vi "fxpAvgSCTL.vi"(7 "reset":bool, 8 "clear":bool, 10 "inputValid":bool=TRUE, 11 "input":fxp<+/-,16,1>) -> (0 "outputValid":bool, 2 "noAvg":u16, 3 "average":fxp<+/-,22,1>, 6 "readyForInput":bool)   [LabVIEW 2016]
uses:
  <vilib>/rvi/FXPMathLib/FxpDiv/subVIs/nifxpmath_Div_SimConfig.ctl
  <vilib>/rvi/FXPMathLib/FxpDiv/simVIs/DllFxpDivTemp_sub.vi
  <vilib>/rvi/FXPMathLib/FxpDiv/XNode/nifxpmath_Div.xnode
  <vilib>/rvi/FXPMathLib/FxpAdd/XNode/nifxpmath_Add.xnode
  <vilib>/rvi/FXPMathLib/sim/FxpSim.dll
panel:
  out "x+y":fxp<+/-,38,16>
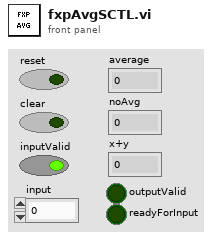
[diagram p1: front panel]
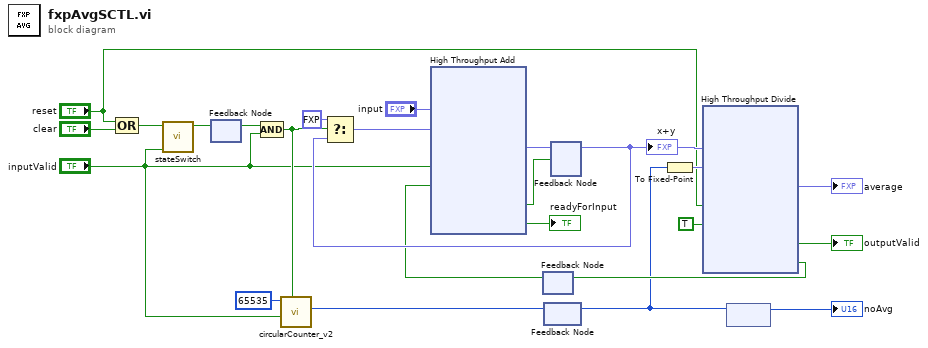
[diagram p0: block diagram]
diagram:
  n1 = Compound Arithmetic op=OR("reset", "clear") -> (w6:bool)
  n2 = call "stateSwitch.vi"("disable"="inputValid", "enable"=w6) -> ("state"=w19:bool)  [unwired: 9 in]
  n3 = feedback #1() -> (w5:bool)  [unwired: 1 in]
  n4 = feedback-in #1(w19) -> ()
  n5 = Compound Arithmetic op=AND(w5, "inputValid") -> (w7:bool)
  n6 = call "circularCounter_v2.vi"("reset"=w7, "doStep"="inputValid", "maxCount"=u16 65535) -> ("next"=w23:u16)  [unwired: 5 in, 3 out]
  n7 = feedback #2() -> (w4:bool)  [unwired: 1 in]
  n8 = feedback #3() -> (w14:u16)  [unwired: 1 in]
  n9 = feedback-in #3(w23) -> ()
  n10 = feedback #4() -> (w13:fxp<+/-,38,16>)  [unwired: 1 in]
  "x+y" <- w13
  n11 = Select(t=fxp<+/-,38,16> 0.0, s=w7, f=w13) -> (s? t:f=w18:fxp<+/-,38,16>)
  n12 = xnode ("High Throughput Add")("x"="input", "y"=w18, "input valid"="inputValid", "ready for output (T)"=w4) -> ("x+y"=w21:fxp<+/-,38,16>, "output valid"=w15:bool, "ready for input"=→"readyForInput":bool)
  n13 = feedback-in #4(w21, w15) -> ()
  n14 = To Fixed-Point(number=w14) -> (fixed-point=w22:fxp<+,16,16>)  [unwired: 1 in]
  n15 = xnode "High Throughput Divide"("x"=w13, "y"=w22, "input valid"="reset", "ready for output (T)"=TRUE) -> ("x/y"=→"average":fxp<+/-,22,1>, "output valid"=→"outputValid":bool, "ready for input"=w20:bool)
  n16 = feedback-in #2(w20) -> ()
  n17 = feedback #5() -> (→"noAvg":u16)  [unwired: 1 in]
  n18 = feedback-in #5(w14) -> ()
